vi "Draw_Cage_Outline_(square).vi"(3 "Error In":errorcluster, 4 "Corner scale  factor":dbl=0.1655 format="%#_13g", 5 "Bounding rectangle for cage outline, pix":T2, 6 "Picture refnum in":T1) -> (0 "Error Out":errorcluster, 2 "Picture refnum out":T1)   [LabVIEW 2018, in "Cage Diagram.lvlib"]
uses:
  Cage Diagram.lvlib
  <vilib>/vision/Image Controls.llb/IMAQ Image.ctl
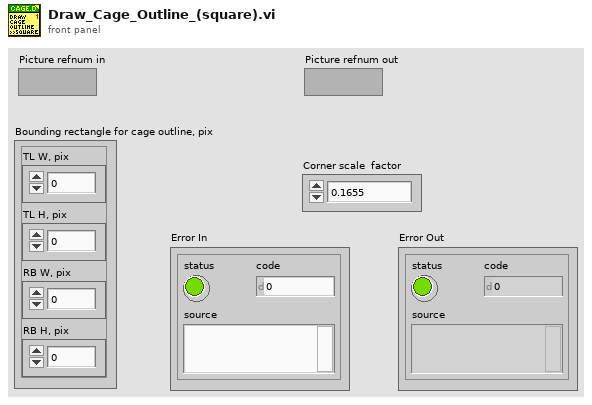
[diagram p1: front panel]
types:
  T1 = typedef "IMAQ Image.ctl" = refnum<image>
  T2 = cluster{"TL W, pix":i32, "TL H, pix":i32, "RB W, pix":i32, "RB H, pix":i32}
  T3 = cluster{"X Left":dbl, "Y Top":dbl, "X Right":dbl, "Y Bottom":dbl}
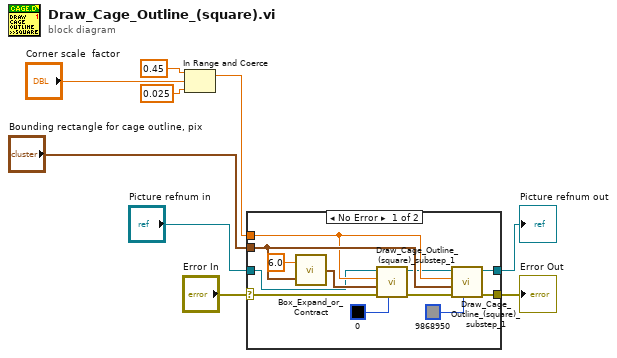
[diagram p0: block diagram]
diagram:
  n1 = In Range and Coerce(upper limit=0.45, x="Corner scale  factor", lower limit=0.025) -> (coerced(x)=w3:dbl)  [unwired: 1 out]
  n2 = case shown="No Error" "Error In" {
    selector: "Error In" -> [w12 w22]
    tunnel: [w13 w23] -> w8
    tunnel: "Picture refnum in" -> [w15 w23]
    tunnel: "Bounding rectangle for cage outline, pix" -> [w21 _]
    tunnel: [w10 w22] -> w5
    tunnel: w3 -> [w18 _]
    frame No Error {
      n3 = call "Box_Expand_or_Contract.vi"("Rectangle in"=w21, "Expand/Contract"=6.0) -> ("Rectangle out"=w19:T3)
      n4 = call "Draw_Cage_Outline_(square)_substep_1.vi"("Color"=u32 0, "error in (no error)"=w12, "Bounding rectangle for cage outline, pix"=w19, "Corner scale  factor"=w18, "Refnum in"=w15) -> ("error out"=w11:errorcluster, "Refnum out"=w14:T1)  [unwired: 5 in]
      n5 = call "Draw_Cage_Outline_(square)_substep_1.vi"("Color"=u32 9868950, "error in (no error)"=w11, "Bounding rectangle for cage outline, pix"=w21, "Corner scale  factor"=w18, "Refnum in"=w14) -> ("error out"=w10:errorcluster, "Refnum out"=w13:T1)  [unwired: 5 in]
    }
    frame Error {
    }
  }
  "Error Out" <- w5
  "Picture refnum out" <- w8
